vi "ReadBackup.vi"(11 "Backup Name":string) -> (0 "error out":errorcluster, 3 "Backup Data":string)   [LabVIEW 2014]
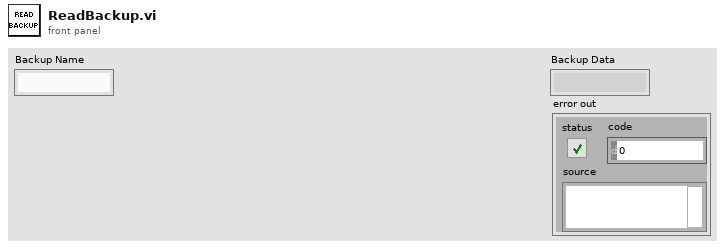
[diagram p1: front panel]
types:
  T1 = enum16{"open", "replace", "create", "open or create", "replace or create", "replace or create with confirmation"}
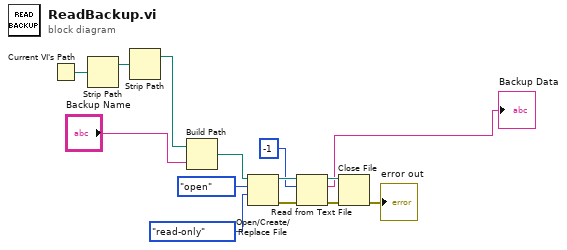
[diagram p0: block diagram]
diagram:
  n1 = Current VI's Path() -> (path=w14:path)
  n2 = Strip Path(path=w14) -> (stripped path=w9:path)  [unwired: 1 out]
  n3 = Strip Path(path=w9) -> (stripped path=w11:path)  [unwired: 1 out]
  n4 = Build Path(base path=w11, name or relative path="Backup Name") -> (appended path=w10:path)
  n5 = Open/Create/Replace File(file path (use dialog)=w10, operation (0:open)=T1."open", access (0:read/write)=enum16{"read/write", "read-only", "write-only"}."read-only") -> (refnum out=w7:refnum<file>, error out=w4:errorcluster)  [unwired: 3 in, 1 out]
  n6 = Read from Text File(file (use dialog)=w7, count=-1, error in=w4) -> (refnum out=w6:refnum<file>, text=→"Backup Data":string, error out=w5:errorcluster)  [unwired: 1 in, 1 out]
  n7 = Close File(refnum=w6, error in=w5) -> (error out=→"error out":errorcluster)  [unwired: 1 out]
